vi "HighlightErrors.vi"(9 "String":string, 10 "Front Panel":refnum<vi>, 11 "Console":refnum<vi>) -> ()   [LabVIEW 2016]
panel:
  out "output cluster":cluster{i32, "offset past match":i32}
  # "Traceback (most recent call last):\n  File \"main.py\", line 56, in <module>\nKeyboardInterrupt:"
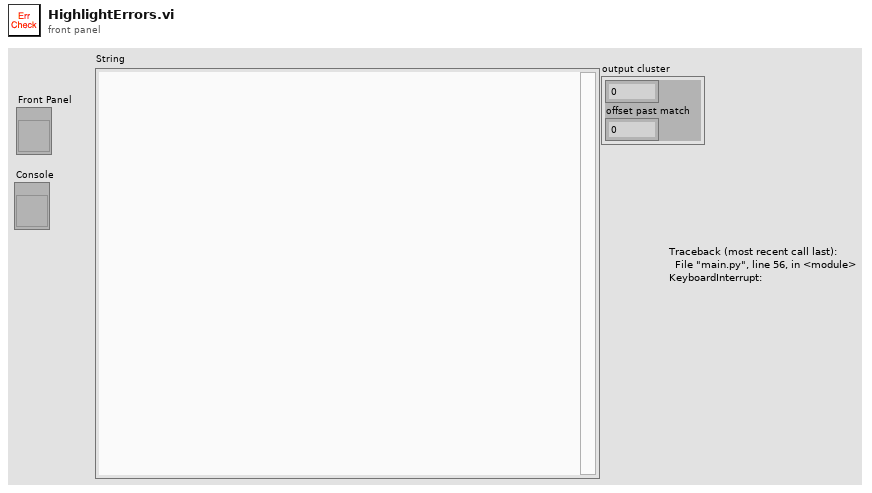
[diagram p1: front panel]
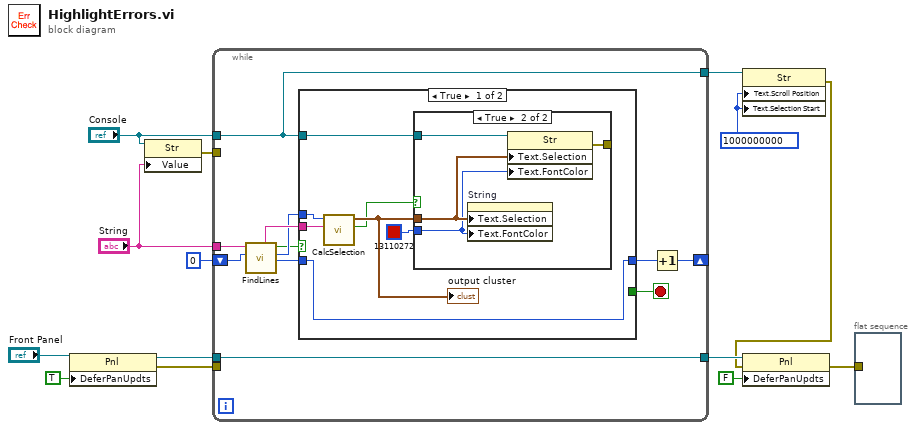
[diagram p0: block diagram]
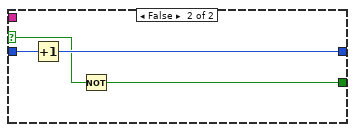
[diagram p3: hidden frame]
diagram:
  w11 = u32 1000000000 ("Text.Selection:Start")
  n1 = property class="Pnl"(reference="Front Panel", "DeferPanUpdts"=TRUE ("Defer Panel Updates")) -> (reference out=w4:refnum<vi>, error out=w2:errorcluster)  [unwired: 1 in]
  n2 = property on="Property Node" class="Str"(reference="Console", "Value"="String") -> (error out=w9:errorcluster)  [unwired: 1 in, 1 out]
  n3 = while {
    tunnel: "String" -> [w24]
    shift-right: [w20] -> _
    shift-left: 0 ("offset past match") -> [w21]
    tunnel: "Console" -> [w19]
    tunnel: [w19] -> w10
    tunnel: w9 -> [_]
    tunnel: [w15] -> w5
    tunnel: w4 -> [w15]
    tunnel: w2 -> [_]
    stop <- w23 stop-if-true
    n4 = call "FindLines.vi"("offset past match in"=w21, "String in"=w24) -> ("Line Number"=w18:i32, "Good?"=w17:bool, "Before"=w25:string, "offset past match out"=w16:i32)  [unwired: 5 in, 1 out]
    n5 = case shown="True" w17 {
      selector: w17 -> [_ w38]
      tunnel: w25 -> [w32 _]
      tunnel: [_ w37] -> w23
      tunnel: [w31 w40] -> w22
      tunnel: w16 -> [w31 w39]
      tunnel: w19 -> [w28 _]
      tunnel: w18 -> [w27 _]
      frame True {
        n6 = call "CalcSelection.vi"("Before"=w32, "Line Number"=w27) -> ("Exists"=w26:bool, "Cluster"=w30:cluster{i32, i32})  [unwired: 8 in]
        "output cluster" <- w30
        n7 = case shown="True" w26 {
          tunnel: w30 -> [_ w36]
          tunnel: u32 13110272 -> [_ w35]
          tunnel: w28 -> [_ w34]
          tunnel: [_ w33] -> _
          frame False {
          }
          frame True {
            n8 = property on="String" class="Str"("Text.Selection"=w36, "Text.FontColor"=w35) -> ()  [unwired: 2 in, 2 out]
            n9 = property on="Property Node" class="Str"(reference=w34, "Text.Selection"=w36, "Text.FontColor"=w35) -> (error out=w33:errorcluster)  [unwired: 1 in, 1 out]
          }
        }
      }
      frame False {
        n10 = Increment(x=w39) -> (x+1=w40:i32)
        n11 = Not(x=w38) -> (.not. x?=w37:bool)
      }
    }
    n12 = Increment(x=w22) -> (x+1=w20:i32)
  }
  n13 = property on="Property Node" class="Str"(reference=w10, "Text.Scroll Position"=w11, "Text.Selection Start"=w11) -> (error out=w3:errorcluster)  [unwired: 1 in, 1 out]
  n14 = property class="Pnl"(reference=w5, error in=w3, "DeferPanUpdts"=FALSE ("Defer Panel Updates")) -> (error out=w1:errorcluster)  [unwired: 1 out]
  n15 = flat-sequence {
    tunnel: w1 -> [_]
    frame #0 {
    }
  }
